vi "Pre-Actor.vi"(8 "error in (no error)":errorcluster, 11 "Instruments in":refnum<class "Instruments.lvclass">) -> (0 "error out":errorcluster, 3 "Instruments out":refnum<class "Instruments.lvclass">)   [LabVIEW 2023, in "Instruments.lvlib" / "Instruments.lvclass"]
doc: "<b>Pre-Actor </b>\nThis routine is called before registering for events, after control references have been mapped to the class private data. It is inteded to perform any additional actions before the actor front panel is displayed.\n\n<b>Instrument</b>\nAt this layer, the engine parent override is removed.\nAt this layer, the instrument calls parse signal list, ancestor classes need to override parse signal list and call parent method of pre-actor if anything needs to be done in addition to parsing signal list."
uses:
  Library/Instruments.lvclass
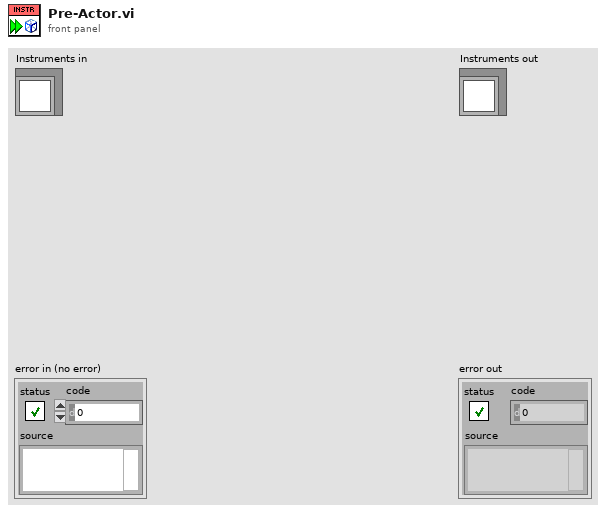
[diagram p1: front panel]
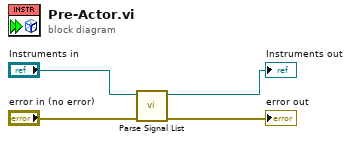
[diagram p0: block diagram]
diagram:
  n1 = call-dynamic "Parse Signal List.vi"("error in (no error)"="error in (no error)", "Configuration in"="Instruments in") -> ("error out"=→"error out":errorcluster, "Configuration out"=→"Instruments out":refnum<class "Instruments.lvclass">)  [unwired: 8 in]
